vi "Think.vi"(8 "Last Direction":T2, 9 "Last Action":T1, 10 "View out":i32[](array[numeric]) caption="Updated View (-1 team, 0 empty, 1 enemy)") -> (1 "Direction":T2, 2 "Action":T1)   [LabVIEW 2017, in "Ant Mound.lvclass"]
uses:
  Ant Mound.lvclass
  Type Defs/Action Enum.ctl
  Type Defs/Direction Enum.ctl
  SubVIs/Read-Only Globals.vi
  SubVIs/Globals (private).vi
  Type Defs/SB Type Defs.lvlib
  DS Square Library/DS Square.lvlib
  Square/Square.lvclass
panel:
  # "NW\nN\nNE\nE\nSE\nS\nSW\nW"
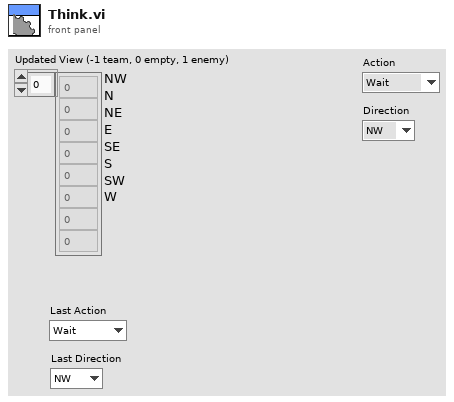
[diagram p1: front panel]
types:
  T1 = typedef "SB Type Defs.lvlib/Action Enum.ctl" = enum16{"Wait", "Move", "Attack", "Replicate"}
  T2 = typedef "SB Type Defs.lvlib/Direction Enum.ctl" = enum16{"NW", "N", "NE", "E", "SE", "S", "SW", "W"}
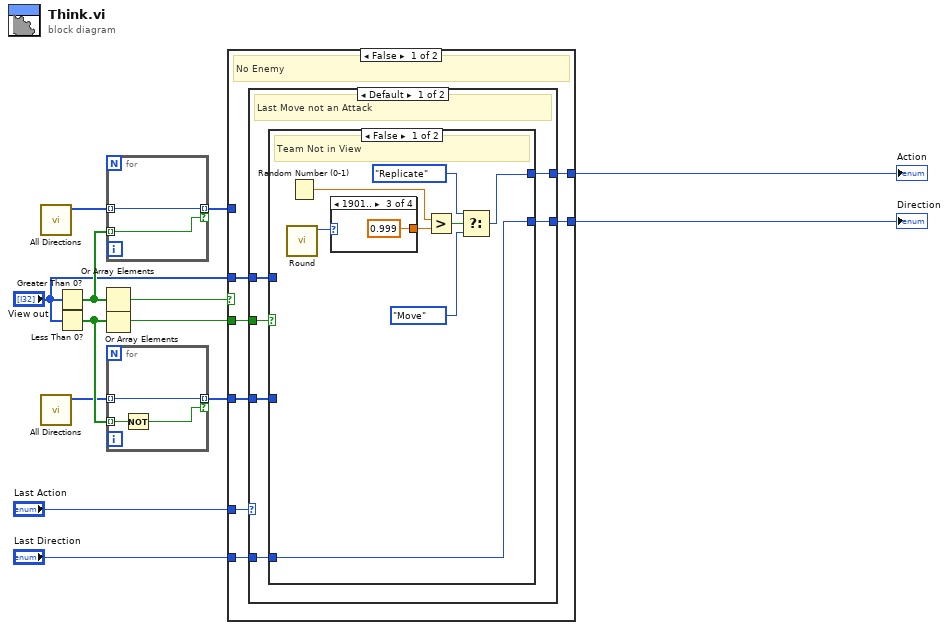
[diagram p0: block diagram]
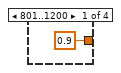
[diagram p2: hidden frame]
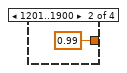
[diagram p3: hidden frame]
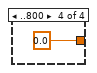
[diagram p4: hidden frame]
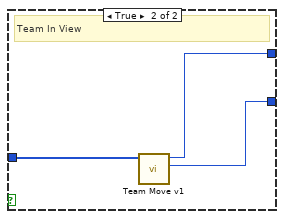
[diagram p5: hidden frame]
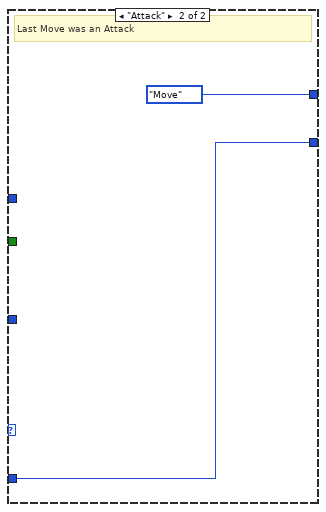
[diagram p6: hidden frame]
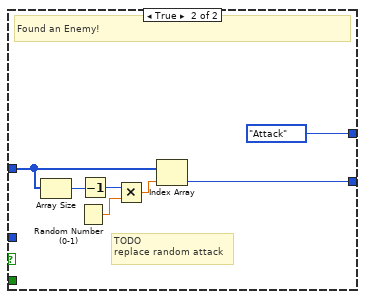
[diagram p7: hidden frame]
diagram:
  n1 = call "All Directions.vi"() -> ("All directions"=w5:T2[])  [unwired: 11 in]
  n2 = call "All Directions.vi"() -> ("All directions"=w4:T2[])  [unwired: 11 in]
  n3 = Greater Than 0?(x="View out") -> (x > 0?=w10:bool[])
  n4 = Less Than 0?(x="View out") -> (x < 0?=w7:bool[])
  n5 = Or Array Elements(Boolean array=w10) -> (logical OR=w9:bool)
  n6 = Or Array Elements(Boolean array=w7) -> (logical OR=w8:bool)
  n7 = for {
    tunnel: w10 -> [w15] mode=indexing
    tunnel: [w14] -> w13 mode=indexing if=w15
    tunnel: w5 -> [w14] mode=indexing
  }
  n8 = for {
    tunnel: w7 -> [w18] mode=indexing
    tunnel: [w16] -> w6 mode=indexing if=w17
    tunnel: w4 -> [w16] mode=indexing
    n9 = Not(x=w18) -> (.not. x?=w17:bool)
  }
  n10 = case shown="False" w9 {
    tunnel: w13 -> [_ w55]
    tunnel: [w23 w50] -> w1
    tunnel: [w24 Action_Enum."Attack" ("Action")] -> w2
    tunnel: "Last Action" -> [w25 _]
    tunnel: "Last Direction" -> [w22 _]
    tunnel: w8 -> [w21 _]
    tunnel: w6 -> [w20 _]
    tunnel: "View out" -> [w19 _]
    frame False {
      # "No Enemy"
      n11 = case shown="Default" w25 {
        tunnel: [w28 Action_Enum."Move" ("Action")] -> w24
        tunnel: [w30 w47] -> w23
        tunnel: w22 -> [w27 w47]
        tunnel: w21 -> [w29 _]
        tunnel: w20 -> [w31 _]
        tunnel: w19 -> [w26 _]
        frame Default {
          # "Last Move not an Attack"
          n12 = case shown="False" w29 {
            tunnel: w31 -> [_ _]
            tunnel: [w39 w44] -> w30
            tunnel: [w34 w45] -> w28
            tunnel: w27 -> [w39 _]
            tunnel: w26 -> [_ w46]
            frame False {
              # "Team Not in View"
              n13 = call "Round.vi"() -> ("Round"=w33:i32)  [unwired: 11 in]
              n14 = Random Number (0-1)() -> (number: 0 to 1=w38:dbl)
              n15 = case shown="1901.." w33 {
                tunnel: [0.9 ("y") 0.99 ("y") 0.999 ("y") 0.0 ("y")] -> w32
                frame 801..1200 {
                }
                frame 1201..1900 {
                }
                frame 1901.. {
                }
                frame ..800 {
                }
              }
              n16 = Greater?(x=w38, y=w32) -> (0:w37:bool)
              n17 = Select(t=Action_Enum."Replicate" ("Action"), s=w37, f=Action_Enum."Move" ("Action")) -> (s? t:f=w34:T1)
            }
            frame True {
              # "Team In View"
              n18 = call "Team Move v1.vi"("View out"=w46) -> ("Direction"=w44:T2, "Action"=w45:T1)  [unwired: 9 in]
            }
          }
        }
        frame "Attack" {
          # "Last Move was an Attack"
        }
      }
    }
    frame True {
      # "TODO\nreplace random attack"
      # "Found an Enemy!"
      n19 = Array Size(array=w55) -> (size(s)=w54:i32)
      n20 = Random Number (0-1)() -> (number: 0 to 1=w52:dbl)
      n21 = Decrement(x=w54) -> (x-1=w53:i32)
      n22 = Multiply(x=w53, y=w52) -> (x*y=w51:dbl)
      n23 = Index Array(array=w55, index=w51) -> (element=w50:T2)
    }
  }
  "Action" <- w2
  "Direction" <- w1
